vi "字符串数组改变解析.vi"(1 "字符串数组":string[](array[string])) -> (14 "删除":string[](array[string]), 16 "新增":string[](array[string]))   [LabVIEW 2019]
uses:
  57a11dd5-0f3c-4e65-926b-2e2e14766b6e.vi
  748c1d5d-bc0b-4984-926a-00e451de2583.vi
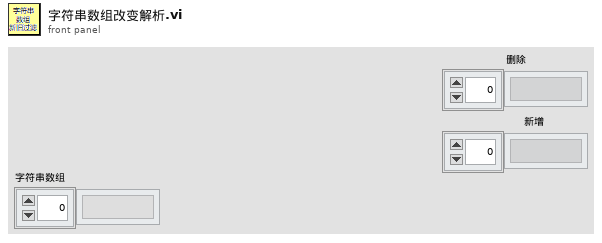
[diagram p1: front panel]
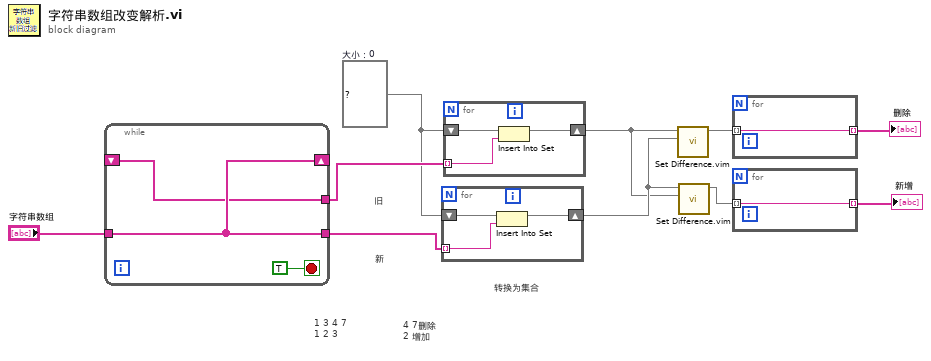
[diagram p0: block diagram]
diagram:
  w7 = set{string} {}  # 大小：0
  # "转换为集合"
  # "4 7删除\n2 增加"
  # "1 3 4 7\n1 2 3"
  # "旧"
  # "新"
  n1 = while {
    tunnel: "字符串数组" -> [w12]
    tunnel: [w12] -> w8
    shift-right: [w12] -> _
    shift-left: _ -> [w11]
    tunnel: [w11] -> w9
    stop <- TRUE stop-if-true
  }
  n2 = for {
    tunnel: w8 -> [w14] mode=indexing
    shift-right: [w15] -> w4
    shift-left: w7 -> [w16]
    n3 = Insert Into Set(10:w14, 11:w16) -> (3:w15:set{string})  [unwired: 1 out]
  }
  n4 = for {
    tunnel: w9 -> [w17] mode=indexing
    shift-right: [w18] -> w3
    shift-left: w7 -> [w19]
    n5 = Insert Into Set(10:w17, 11:w19) -> (3:w18:set{string})  [unwired: 1 out]
  }
  n6 = call "Set Difference.vim"("set 2"=w4, "set 1"=w3) -> ("difference"=w6:set{string})  [unwired: 9 in]
  n7 = call "Set Difference.vim"("set 2"=w3, "set 1"=w4) -> ("difference"=w2:set{string})  [unwired: 9 in]
  n8 = for {
    tunnel: [w20] -> w5 mode=indexing
    tunnel: w6 -> [w20] mode=indexing
  }
  "删除" <- w5
  n9 = for {
    tunnel: [w21] -> w1 mode=indexing
    tunnel: w2 -> [w21] mode=indexing
  }
  "新增" <- w1
